vi "Get Resource.vi"(8 "error in (no error)":errorcluster, 11 "Device in":refnum<class "Device.lvclass">) -> (0 "error out":errorcluster, 2 "Resource":refnum<class "Resource.lvclass">, 3 "Device out":refnum<class "Device.lvclass">)   [LabVIEW 2020, in "PicoG-App.lvlib" / "Device.lvclass"]
uses:
  Device.lvclass
  Builds/picoG/ppl/PicoG-Core.lvlibp/PicoG-Processor/PicoG-Core/Resource/Resource.lvclass
  Device.lvclass/Device.ctl
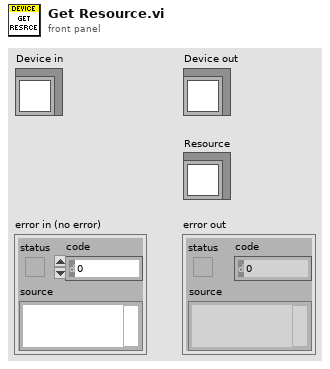
[diagram p1: front panel]
types:
  T1 = typedef "PicoG-App.lvlib/Device.lvclass/Resource Ref.ctl" = cluster{"Resource":refnum<class "Resource.lvclass">, "Open":bool, "At Prompt":bool, "Running":bool}
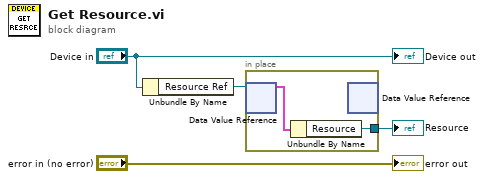
[diagram p0: block diagram]
diagram:
  n1 = Unbundle By Name("Device in") -> ("Resource Ref"=w3:refnum<data-value>)
  n2 = in-place {
    in-place-border: [w5] -> w1
    n3 = in-place-dvr #1(w3) -> (w6:T1)  [unwired: 1 out]
    n4 = Unbundle By Name(w6) -> ("Resource"=w5:refnum<class "Resource.lvclass">)
    n5 = in-place-dvr #1() -> ()  [unwired: 1 in, 2 out]
  }
  "Resource" <- w1
  "error out" <- "error in (no error)"
  "Device out" <- "Device in"
